vi "Display and Log Custom Device Error.vi"(8 "error out":errorcluster, 9 "Note (empty)":string, 10 "Your code's public name":string, 11 "Custom Device? (T)":bool=TRUE) -> ()   [LabVIEW 2015, in "VS Inline Async API.lvlib" / "VS Inline Async API.lvclass"]
uses:
  VS Inline Async API.lvclass
  <vilib>/NI Veristand/Custom Device Tools/Custom Device Utility Library/Custom Device Utility Library.lvlib
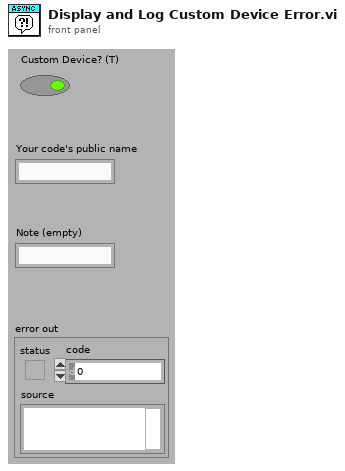
[diagram p1: front panel]
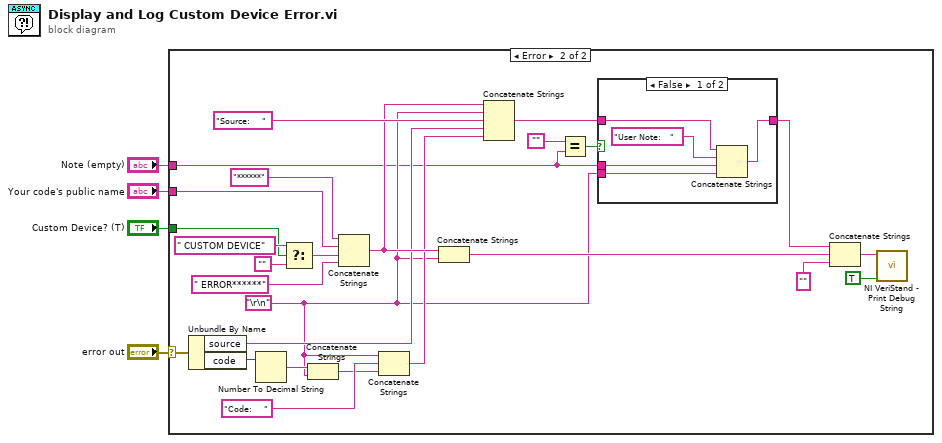
[diagram p0: block diagram]
diagram:
  n1 = case shown="Error" "error out" {
    selector: "error out" -> [_ w30]
    tunnel: "Custom Device? (T)" -> [_ w18]
    tunnel: "Your code's public name" -> [_ w9]
    tunnel: "Note (empty)" -> [_ w7]
    frame No Error {
    }
    frame Error {
      w8 = "\r\n"
      n2 = Unbundle By Name(w30) -> ("source"=w17:string, "code"=w11:i32)
      n3 = Number To Decimal String(number=w11) -> (decimal integer string=w27:string)  [unwired: 1 in]
      n4 = Select(t=" CUSTOM DEVICE" ("String"), s=w18, f="") -> (s? t:f=w19:string)
      n5 = Concatenate Strings(w27, w8) -> (w10:string)
      n6 = Concatenate Strings("******" ("String"), w9, w19, " ERROR******" ("String")) -> (w22:string)
      n7 = Concatenate Strings(w8, "Code:    " ("String"), w10) -> (w16:string)
      n8 = Concatenate Strings(w22, w8) -> (w13:string)
      n9 = Concatenate Strings(w22, w8, "Source:    " ("String"), w17, w16) -> (w15:string)
      n10 = Equal?(x="", y=w7) -> (x = y?=w20:bool)
      n11 = case shown="False" w20 {
        tunnel: w7 -> [w34 _]
        tunnel: w8 -> [w33 _]
        tunnel: w15 -> [w32 w36]
        tunnel: [w31 w36] -> w14
        frame False {
          n12 = Concatenate Strings(w32, "User Note:   " ("string"), w34, w33) -> (w31:string)
        }
        frame True {
        }
      }
      n13 = Concatenate Strings(w14, w13, "" ("Message")) -> (w6:string)
      n14 = call <vilib>:"NI VeriStand - Print Debug String.vi"("Add to log file? (T)"=TRUE, "Message"=w6) -> ()  [unwired: 9 in, 1 out]
    }
  }
